vi "GPSCoorTrans(SubVI).vi"(9 "Height":dbl format="%#_13g", 10 "Longitude":dbl format="%#_13g", 11 "Latitude":dbl format="%#_13g") -> (3 "Output":dbl[](array[numeric])=[-92.50930918799867, 134.61356086615828, -0.002149326671514001])   [LabVIEW 2019]
uses:
  <vilib>/Analysis/Matrix/Numeric/Conversions/Array To Matrix - RA.vi
  <vilib>/Analysis/Matrix/Numeric/Conversions/Array To Matrix - RA2.vi
  <vilib>/Analysis/Matrix/Numeric/Multiply/Multiply - RM,RM.vi
  <vilib>/Analysis/Matrix/Numeric/Conversions/Matrix To Array - RM.vi
  <vilib>/Analysis/Matrix/NI_Matrix.lvlib
panel:
  out "N":dbl=6385650.46895231 format="%#_19f"
  out "cos(phi)":dbl=0.8054084671539502
  out "sin(phi)":dbl=0.5927201709379599
  out "sin(lam)":dbl=0.7945576903808257
  out "cos(lam)":dbl=-0.607188666442884
  out "b^2/a^2":dbl=0.9933056200098537
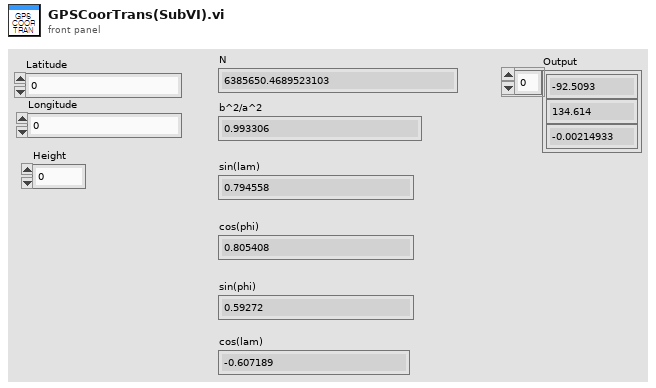
[diagram p1: front panel]
types:
  T1 = typedef "NI_Matrix.lvlib/RealMatrix.ctl" = dbl[][]
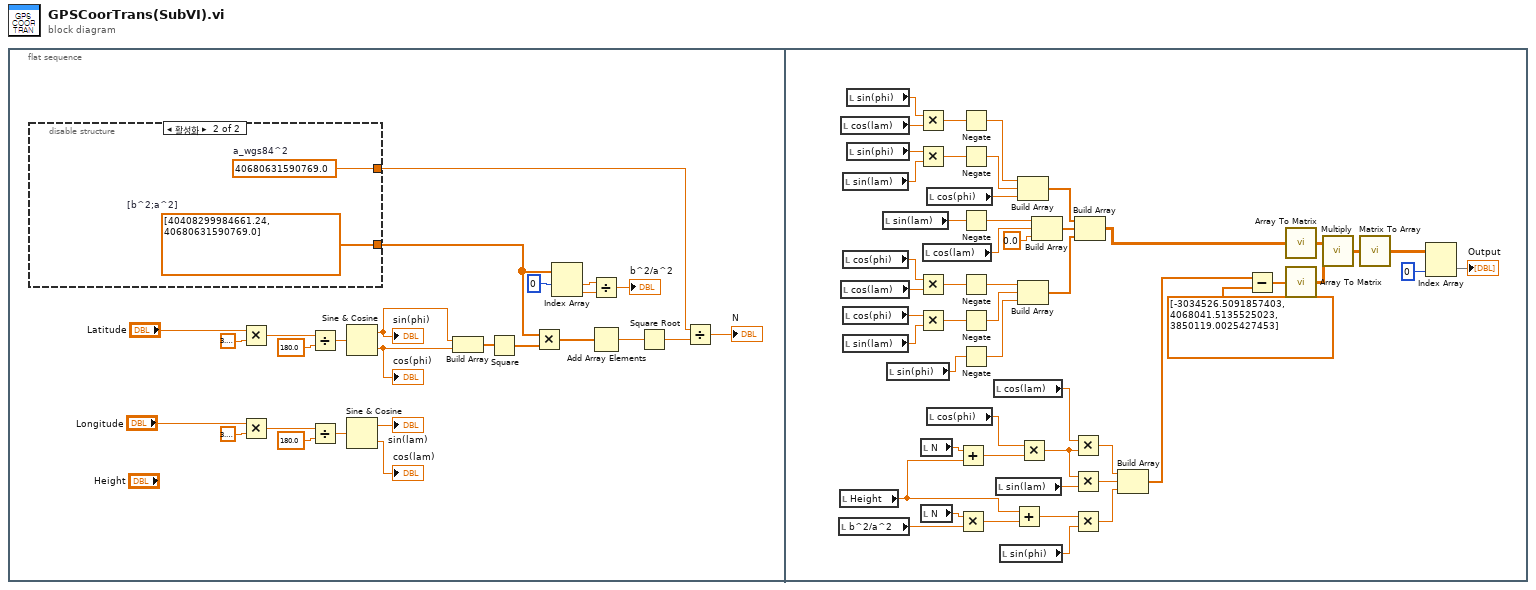
[diagram p0: block diagram]
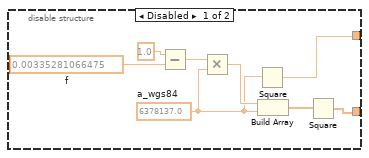
[diagram p2: hidden frame]
diagram:
  n1 = flat-sequence {
    frame #0 {
      n2 = disable-structure shown="활성화" {
        disable-tunnel: [w29 w36] -> w1
        disable-tunnel: [w27 w35] -> w2
        frame Disabled {
          w34 = 0.00335281066475  # f
          w28 = 6378137.0  # a_wgs84
          n3 = Subtract(x=1.0, y=w34) -> (x-y=w32:dbl)
          n4 = Multiply(x=w32, y=w28) -> (x*y=w31:dbl)
          n5 = Square(x=w28) -> (x^2=w27:dbl)
          n6 = Build Array(w31, w28) -> (w30:dbl[])
          n7 = Square(x=w30) -> (x^2=w29:dbl[])
        }
        frame Enabled {
          w35 = 40680631590769.0  # a_wgs84^2
          w36 = dbl[] [40408299984661.24, 40680631590769.0]  # [b^2;a^2]
        }
      }
      n8 = Multiply(x="Latitude", y=3.141592653589793) -> (x*y=w7:dbl)
      n9 = Multiply(x="Longitude", y=3.141592653589793) -> (x*y=w23:dbl)
      n10 = Divide(x=w7, y=180.0) -> (x/y=w9:dbl)
      n11 = Divide(x=w23, y=180.0) -> (x/y=w21:dbl)
      n12 = Sine & Cosine(0:w9) -> (1:w10:dbl, 2:w11:dbl)
      "sin(phi)" <- w10
      "cos(phi)" <- w11
      n13 = Sine & Cosine(0:w21) -> (1:→"sin(lam)":dbl, 2:→"cos(lam)":dbl)
      n14 = Build Array(w10, w11) -> (w12:dbl[])
      n15 = Square(x=w12) -> (x^2=w13:dbl[])
      n16 = Multiply(x=w1, y=w13) -> (x*y=w16:dbl[])
      n17 = Index Array(array=w1, index #1=0 ("index")) -> (element #1=w18:dbl, element #2=w19:dbl)  [unwired: 1 in]
      n18 = Divide(x=w18, y=w19) -> (x/y=→"b^2/a^2":dbl)
      n19 = Add Array Elements(numeric array=w16) -> (sum=w14:dbl)
      n20 = Square Root(x=w14) -> (sqrt(x)=w15:dbl)
      n21 = Divide(x=w2, y=w15) -> (x/y=→"N":dbl)
    }
    frame #1 {
      n22 = local read "b^2/a^2"() -> (w77:dbl)
      n23 = local read "Height"() -> (w80:dbl)
      n24 = local read "cos(lam)"() -> (w71:dbl)
      n25 = local read "cos(lam)"() -> (w53:dbl)
      n26 = local read "sin(lam)"() -> (w68:dbl)
      n27 = local read "cos(phi)"() -> (w52:dbl)
      n28 = local read "cos(phi)"() -> (w57:dbl)
      n29 = local read "sin(lam)"() -> (w56:dbl)
      n30 = local read "sin(phi)"() -> (w72:dbl)
      n31 = local read "sin(phi)"() -> (w67:dbl)
      n32 = local read "sin(lam)"() -> (w63:dbl)
      n33 = local read "sin(phi)"() -> (w51:dbl)
      n34 = Multiply(x=w72, y=w71) -> (x*y=w70:dbl)
      n35 = Multiply(x=w67, y=w68) -> (x*y=w69:dbl)
      n36 = Multiply(x=w52, y=w53) -> (x*y=w54:dbl)
      n37 = Multiply(x=w57, y=w56) -> (x*y=w55:dbl)
      n38 = local read "N"() -> (w79:dbl)
      n39 = local read "N"() -> (w78:dbl)
      n40 = local read "cos(lam)"() -> (w61:dbl)
      n41 = local read "cos(phi)"() -> (w64:dbl)
      n42 = local read "cos(phi)"() -> (w75:dbl)
      n43 = Add(x=w79, y=w80) -> (x+y=w87:dbl)
      n44 = Multiply(x=w78, y=w77) -> (x*y=w83:dbl)
      n45 = Negate(x=w70) -> (-x=w66:dbl)
      n46 = Negate(x=w69) -> (-x=w65:dbl)
      n47 = Negate(x=w63) -> (-x=w62:dbl)
      n48 = Negate(x=w54) -> (-x=w58:dbl)
      n49 = Negate(x=w55) -> (-x=w59:dbl)
      n50 = Negate(x=w51) -> (-x=w50:dbl)
      n51 = local read "cos(lam)"() -> (w74:dbl)
      n52 = local read "sin(lam)"() -> (w73:dbl)
      n53 = local read "sin(phi)"() -> (w76:dbl)
      n54 = Add(x=w80, y=w83) -> (x+y=w82:dbl)
      n55 = Build Array(w66, w65, w64) -> (w49:dbl[])
      n56 = Build Array(w58, w59, w50) -> (w47:dbl[])
      n57 = Multiply(x=w75, y=w87) -> (x*y=w86:dbl)
      n58 = Build Array(w62, w61, 0.0 ("element")) -> (w48:dbl[])
      n59 = Multiply(x=w74, y=w86) -> (x*y=w85:dbl)
      n60 = Multiply(x=w86, y=w73) -> (x*y=w84:dbl)
      n61 = Multiply(x=w82, y=w76) -> (x*y=w81:dbl)
      n62 = Build Array(w49, w48, w47) -> (w39:dbl[][])
      n63 = Build Array(w85, w84, w81) -> (w38:dbl[])
      n64 = Subtract(x=w38, y=dbl[] [-3034526.5091857403, 4068041.5135525023, 3850119.0025427453] ("ECEF ref")) -> (x-y=w45:dbl[])
      n65 = call-poly <vilib>:"Array To Matrix.vi"("Real 2D Array"=w39) -> ("Real Matrix"=w44:T1)
      n66 = call-poly <vilib>:"Array To Matrix.vi"("Real 1D Array"=w45) -> ("Real Matrix (Column Vector)"=w46:T1)
      n67 = call-poly <vilib>:"Multiply.vi"("Real Matrix B"=w46, "Real Matrix A"=w44) -> ("A * B"=w42:T1)
      n68 = call-poly <vilib>:"Matrix To Array.vi"("Real Matrix"=w42) -> ("Real 2D Array"=w43:dbl[][])
      n69 = Index Array(array=w43, index (col)=0 ("disabled index (col)")) -> (element=→"Output":dbl[])  [unwired: 1 in]
    }
  }
